vi "Main Page.vi"(8 "error in (no error)":errorcluster, 11 "Node Ptr":T1 format="%.0x") -> (0 "error out":errorcluster)   [LabVIEW 2015, in "Waveform-Processing-Custom-Device System Explorer.lvlib"]
uses:
  Waveform-Processing-Custom-Device System Explorer.lvlib
  <vilib>/NI Veristand/Custom Device API/Custom Device Item Ref.ctl
  Shared/Types/FG Action.ctl
  Types/UI Refs Ctl.ctl
  Shared/Constants.vi
  <vilib>/NI Veristand/Custom Device API/Set Item Property (Boolean).vi
  <vilib>/NI VeriStand/Custom Device API/Custom Device API.lvlib
  Shared/Waveform-Processing-Custom-Device Shared.lvlib
  Shared/Running Average/Running Average.lvlib
  Shared/Single Point/SinglePoint.lvlib
  Shared/Scaled Waveform/Scaled Waveform.lvlib
panel:
  in  "Scaled Waveform":bool
  in  "Header 2":cluster{"Section Name":string}={"Section Name"="Custom Device Item Settings"}
  out "Task Rate (Hz)":dbl
  in  "Buffer Length (s)":dbl format="%#_6f"
  out "Buffer Length (samples)":u32
  in  "Description":string
  in  "Remove Channel":bool
  in  "Add Channel":bool
  in  "Selected Waveforms":i32[](listbox)
  in  "Waveform Task":u16(ring) items=["Waveform1"=11, "Waveform2"=15]
  in  "Available Waveforms":i32[](listbox)
  in  "Single-point":bool
  in  "Running Average":bool
  in  "Header":cluster{"Section Name":string}={"Section Name"="Custom Device Item Settings"}
  in  "Name":string
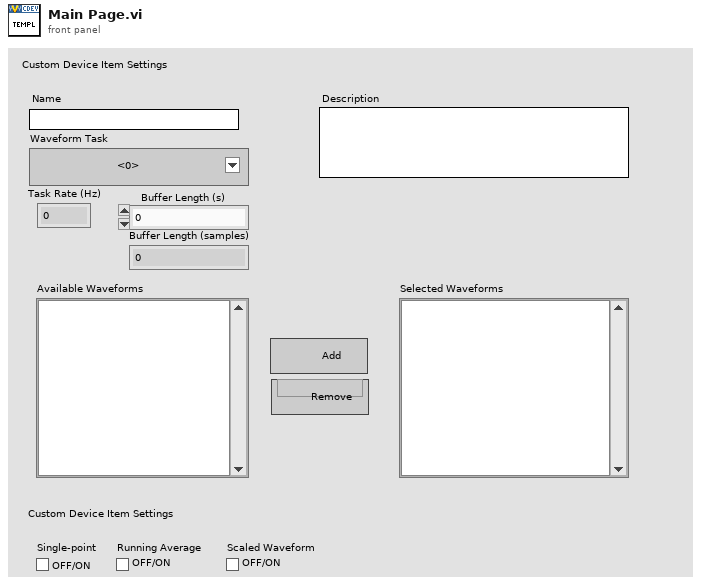
[diagram p1: front panel]
types:
  T1 = typedef "Custom Device API.lvlib/Custom Device Item Ref.ctl" = u64
  T2 = typedef "Waveform-Processing-Custom-Device Shared.lvlib/UI Refs Ctl.ctl" = cluster{"Selected Waveforms":refnum<vi>, "Available Waveforms":refnum<vi>, "Wfm Task Rate (Hz)":refnum<vi>, "Buffer Length (s)":refnum<vi>, "Buffer Length (samples)":refnum<vi>, "Add Channel":refnum<vi>, "Remove Channel":refnum<vi>, "Running Average":refnum<vi>, "Single-point":refnum<vi>, "Waveform Task":refnum<vi>, "Scaled Waveform":refnum<vi>}
  T3 = typedef "Waveform-Processing-Custom-Device Shared.lvlib/FG Action.ctl" = enum8{"GET", "SET"}
  T4 = typedef "Custom Device API.lvlib/Custom Device Item Info.ctl" = cluster{"Name":string, "Is Channel":bool, "GUID":string, "Is Waveform":bool}
  T5 = typedef "Waveform-Processing-Custom-Device Shared.lvlib/Custom Device Settings.ctl" = cluster{"CD Task Dependency":T1, "CD Task Dependency Ref":T1, "CD Task Available Wfms":string[], "CD Task Selected Wfms":string[], "Buffer Length (s)":dbl, "Buffer Length (samples)":u32, "Task Rate":dbl, "Single-point Enabled":bool, "Running Average Enabled":bool, "Scaled Waveform Enabled":bool}
  T6 = typedef "Custom Device API.lvlib/Custom Device Commands.ctl" = enum16{"Default", "Item renamed", "Shutdown", "Dynamic button pressed"}
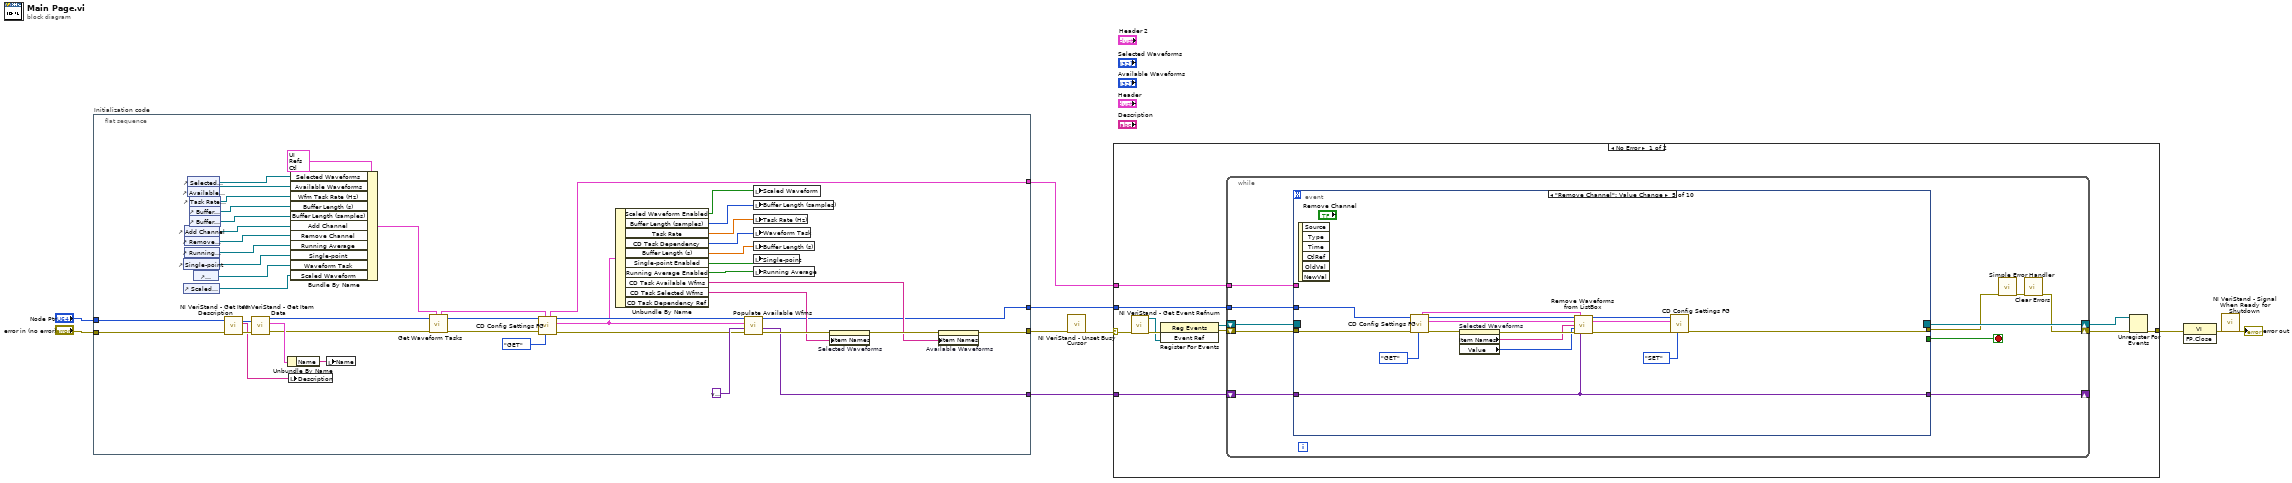
[diagram p0: block diagram]
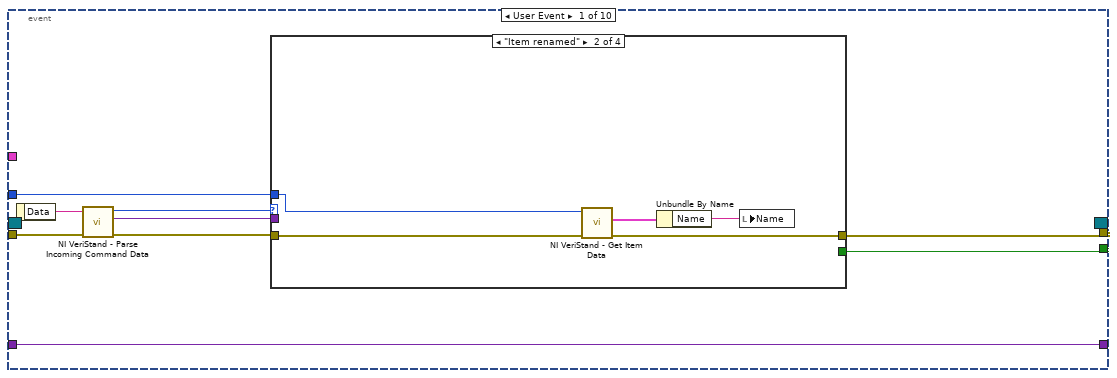
[diagram p2: hidden frame]
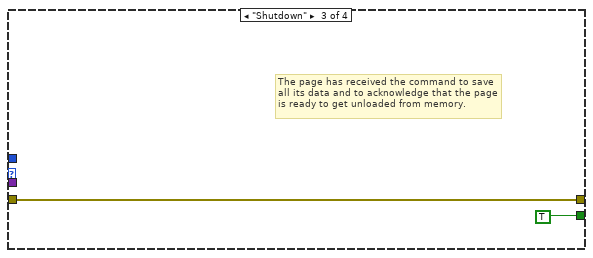
[diagram p4: hidden frame]
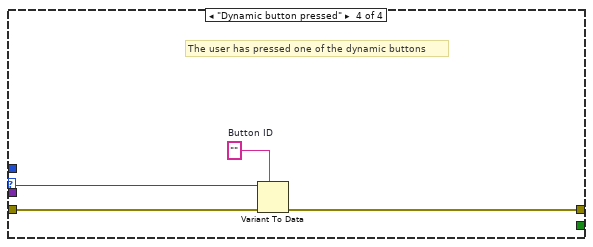
[diagram p5: hidden frame]
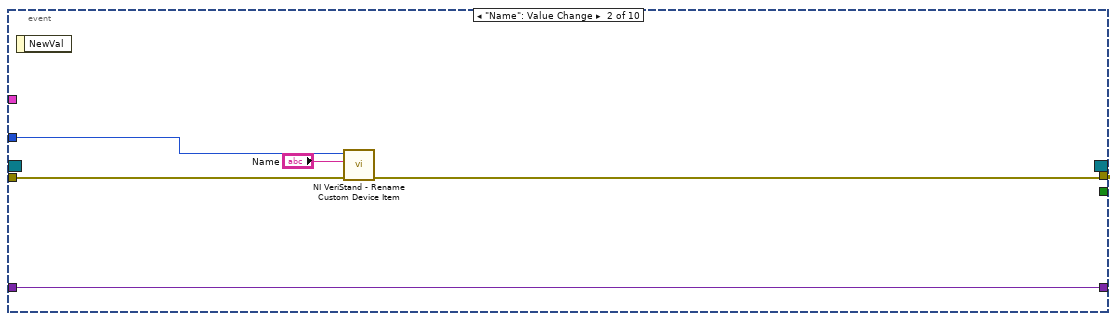
[diagram p6: hidden frame]
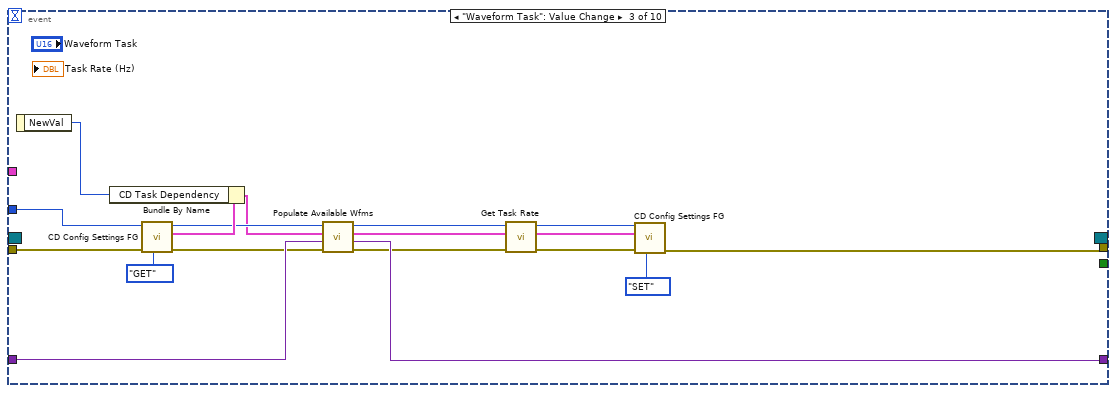
[diagram p7: hidden frame]
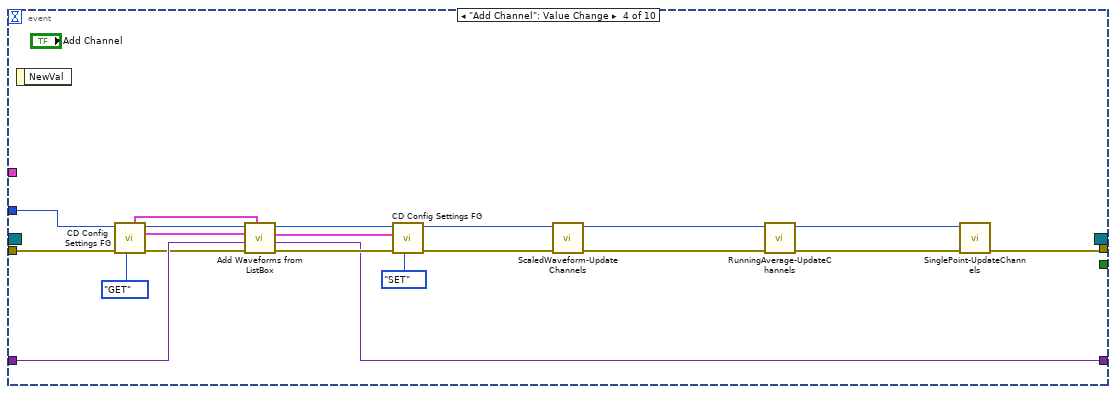
[diagram p8: hidden frame]
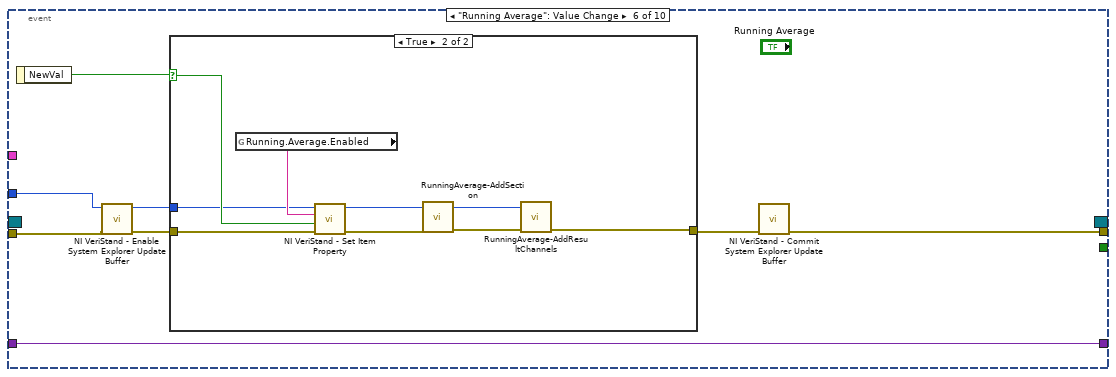
[diagram p9: hidden frame]
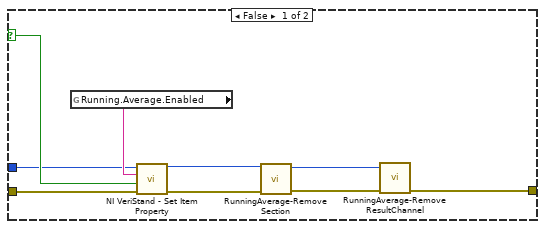
[diagram p10: hidden frame]
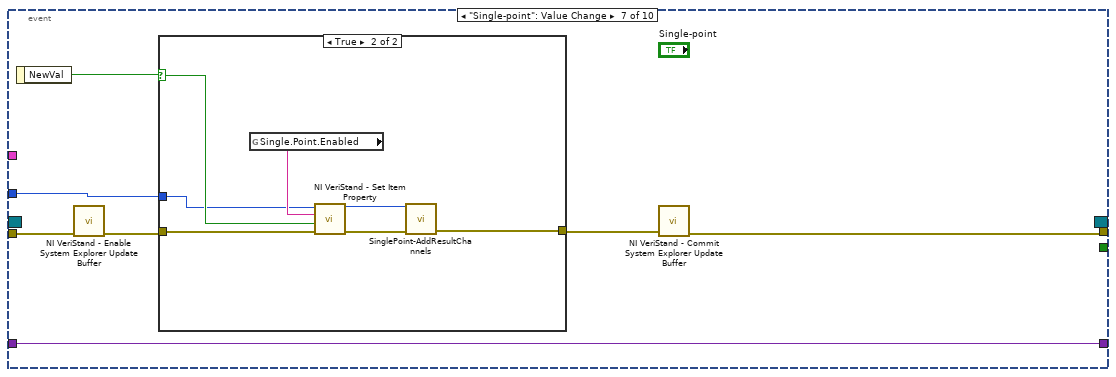
[diagram p11: hidden frame]
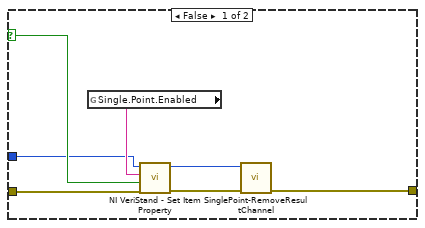
[diagram p12: hidden frame]
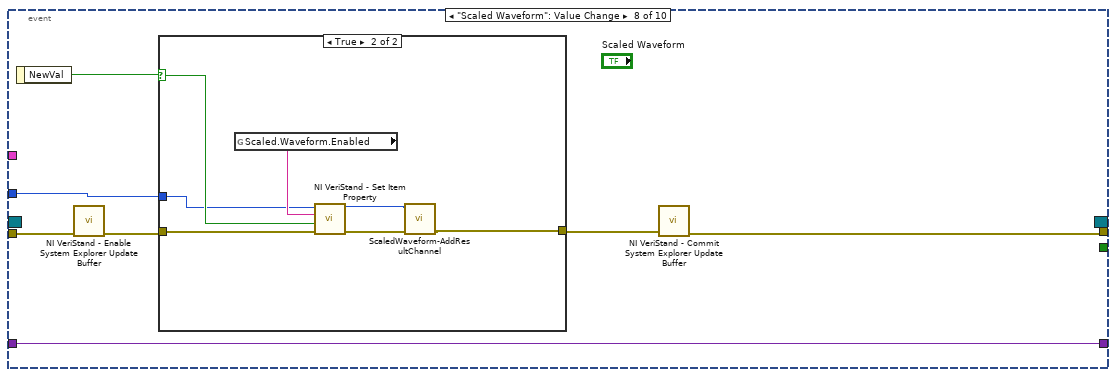
[diagram p13: hidden frame]
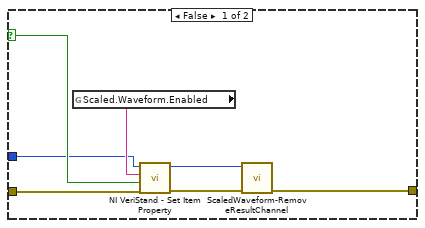
[diagram p14: hidden frame]
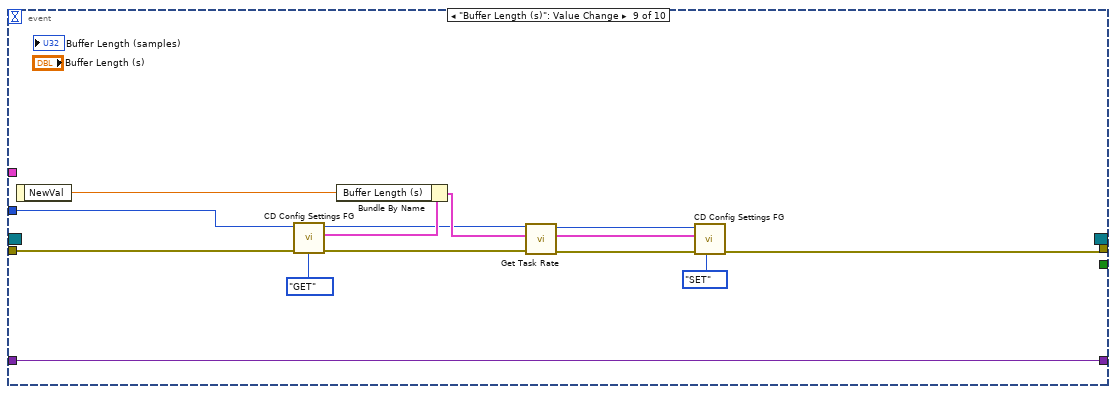
[diagram p15: hidden frame]
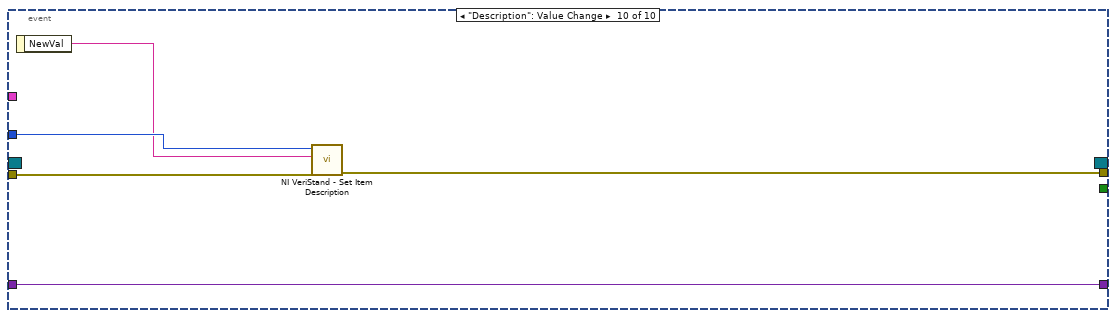
[diagram p16: hidden frame]
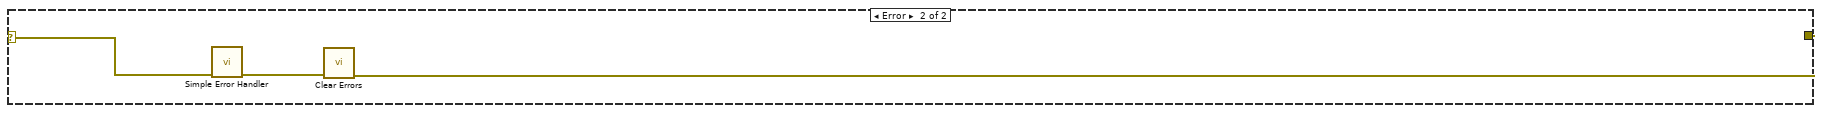
[diagram p17: hidden frame]
diagram:
  n1 = flat-sequence "Initialization code" {
    tunnel: "error in (no error)" -> [w54]
    tunnel: "Node Ptr" -> [w53]
    tunnel: [w40] -> w1
    tunnel: [w17] -> w4
    tunnel: [w15] -> w3
    tunnel: [w18] -> w2
    frame #0 {
      n2 = control-ref of="Single-point"() -> (w37:refnum<vi>)
      n3 = control-ref of="Scaled Waveform"() -> (w12:refnum<vi>)
      n4 = control-ref of="Add Channel"() -> (w34:refnum<vi>)
      n5 = control-ref of="Remove Channel"() -> (w35:refnum<vi>)
      n6 = control-ref of="Running Average"() -> (w36:refnum<vi>)
      n7 = control-ref of="Selected Waveforms"() -> (w29:refnum<vi>)
      n8 = control-ref of="Available Waveforms"() -> (w30:refnum<vi>)
      n9 = control-ref of="Task Rate (Hz)"() -> (w31:refnum<vi>)
      n10 = control-ref of="Buffer Length (s)"() -> (w32:refnum<vi>)
      n11 = control-ref of="Buffer Length (samples)"() -> (w33:refnum<vi>)
      n12 = control-ref of="Waveform Task"() -> (w19:refnum<vi>)
      n13 = call <vilib>:"NI VeriStand - Get Item Description.vi"("error in (no error)"=w54, "Item Ref in"=w53) -> ("error out"=w52:errorcluster, "Description"=w49:string, "Item Ref out"=w55:T1)  [unwired: 7 out]
      n14 = call <vilib>:"NI VeriStand - Get Item Data.vi"("error in (no error)"=w52, "Item Ref in"=w55) -> ("error out"=w26:errorcluster, "Item Info"=w51:T4, "Item Ref out"=w20:T1)  [unwired: 7 out]
      n15 = Unbundle By Name(w51) -> ("Name"=w50:string)
      n16 = local write "Description"(w49) -> ()
      n17 = Bundle By Name(cluster=T2 {"Selected Waveforms"=refnum, "Available Waveforms"=refnum, "Wfm Task Rate (Hz)"=refnum, "Buffer Length (s)"=refnum, "Buffer Length (samples)"=refnum, "Add Channel"=refnum, "Remove Channel"=refnum, "Running Average"=refnum, "Single-point"=refnum, "Waveform Task"=refnum, "Scaled Waveform"=refnum} ("UI Refs"), "Selected Waveforms"=w29, "Available Waveforms"=w30, "Wfm Task Rate (Hz)"=w31, "Buffer Length (s)"=w32, "Buffer Length (samples)"=w33, "Add Channel"=w34, "Remove Channel"=w35, "Running Average"=w36, "Single-point"=w37, "Waveform Task"=w19, "Scaled Waveform"=w12) -> (w25:T2)
      n18 = local write "Name"(w50) -> ()
      n19 = call "Get Waveform Tasks.vi"("Custom Device ref in"=w20, "error in"=w26, "UI Refs in"=w25) -> ("UI Refs out"=w24:T2, "Custom Device ref out"=w23:T1, "error out"=w27:errorcluster)  [unwired: 5 in]
      n20 = call "CD Config Settings FG.vi"("Action"=FG_Action."GET", "UI Refs"=w24, "error in (no error)"=w27, "Item Ref"=w23) -> ("error out"=w22:errorcluster, "CD Settings out"=w13:T5, "Item Ref out"=w21:T1, "UI Refs out"=w18:T2)  [unwired: 4 in]
      n21 = Unbundle By Name(w13) -> ("Scaled Waveform Enabled"=w11:bool, "Buffer Length (samples)"=w14:u32, "Task Rate"=w16:dbl, "CD Task Dependency"=w28:T1, "Buffer Length (s)"=w46:dbl, "Single-point Enabled"=w48:bool, "Running Average Enabled"=w47:bool, "CD Task Available Wfms"=w41:string[], "CD Task Selected Wfms"=w42:string[])  [unwired: 1 out]
      n22 = call "Populate Available Wfms.vi"("error in"=w22, "ListBox Variant"=variant, "CD Settings"=w13, "CustomDevice Ref"=w21) -> ("error out"=w44:errorcluster, "ListBox Variant"=w40:variant, "CustomDevice Ref"=w15:T1)  [unwired: 4 in, 1 out]
      n23 = local write "Scaled Waveform"(w11) -> ()
      n24 = local write "Buffer Length (samples)"(w14) -> ()
      n25 = local write "Task Rate (Hz)"(w16) -> ()
      n26 = local write "Waveform Task"(w28) -> ()
      n27 = local write "Buffer Length (s)"(w46) -> ()
      n28 = local write "Single-point"(w48) -> ()
      n29 = local write "Running Average"(w47) -> ()
      n30 = property on="Selected Waveforms" class="LstBox (strict)"(error in=w44, "Item Names"=w42) -> (error out=w43:errorcluster)  [unwired: 1 in, 1 out]
      n31 = property on="Available Waveforms" class="LstBox (strict)"(error in=w43, "Item Names"=w41) -> (error out=w17:errorcluster)  [unwired: 1 in, 1 out]
    }
  }
  n32 = call <vilib>:"NI VeriStand - Unset Busy Cursor.vi"("error in (no error)"=w4) -> ("error out"=w6:errorcluster)  [unwired: 10 out]
  n33 = case shown="No Error" w6 {
    selector: w6 -> [w59 w246]
    tunnel: [w63 w244] -> w10
    tunnel: w3 -> [w58 _]
    tunnel: w1 -> [w57 _]
    tunnel: w2 -> [w56 _]
    frame No Error {
      n34 = call <vilib>:"NI VeriStand - Get Event Refnum.vi"("error in (no error)"=w59) -> ("error out"=w66:errorcluster, "Event Ref"=w62:refnum<user-event>)  [unwired: 9 out]
      n35 = register-events(error in=w66, w62) -> (reference out=w60:refnum<event-registration>, error out=w61:errorcluster)  [unwired: 1 in]
      n36 = while {
        shift-right: [w73] -> w64
        shift-left: w61 -> [w69]
        shift-right: [w77] -> w65
        shift-left: w60 -> [w76]
        tunnel: w58 -> [w72]
        shift-right: [w71] -> _
        shift-left: w57 -> [w70]
        tunnel: w56 -> [w67]
        stop <- w75 stop-if-true
        n37 = event shown="[4] \"Remove Channel\": Value Change" {
          selector: w76 -> [_ _ _ _ _ _ _ _ _ _]
          dyn-events: [_ _ _ _ _ _ _ _ _ _] -> w77
          timeout: _ -> [_ _ _ _ _ _ _ _ _ _]
          tunnel: w69 -> [w86 w103 w118 w135 w154 w161 w186 w207 w237 w243]
          tunnel: [w82 _ _ _ _ _ _ _ _ _] -> w75
          tunnel: [w81 w102 w104 w131 w143 w158 w183 w204 w225 w242] -> w68
          tunnel: w72 -> [w79 w100 w117 w141 w157 w163 w188 w209 w235 w241]
          tunnel: [w78 w99 w121 w127 w142 w162 w187 w208 w238 w239] -> w71
          tunnel: w70 -> [w78 w99 w120 w129 w142 w162 w187 w208 w238 w239]
          tunnel: w67 -> [_ _ _ _ _ _ _ _ _ _]
          event User Event {
            n38 = event-data() -> ("Data"=w85:string)  [unwired: 1 out]
            n39 = call <vilib>:"NI VeriStand - Parse Incoming Command Data.vi"("error in (no error)"=w86, "Incoming data"=w85) -> ("error out"=w84:errorcluster, "Outgoing data"=w80:variant, "Action"=w83:T6)  [unwired: 7 out]
            n40 = case shown="\"Item renamed\"" w83 {
              tunnel: w84 -> [w87 w92 w93 w98]
              tunnel: [_ _ TRUE _] -> w82
              tunnel: [w87 w90 w93 w95] -> w81
              tunnel: w80 -> [_ _ _ w97]
              tunnel: w79 -> [_ w88 _ _]
              frame "Default", Default {
              }
              frame "Item renamed" {
                n41 = call <vilib>:"NI VeriStand - Get Item Data.vi"("error in (no error)"=w92, "Item Ref in"=w88) -> ("error out"=w90:errorcluster, "Item Info"=w91:T4)  [unwired: 8 out]
                n42 = Unbundle By Name(w91) -> ("Name"=w89:string)
                n43 = local write "Name"(w89) -> ()
              }
              frame "Shutdown" {
                # "The page has received the command to save all its data and to acknowledge that the page is ready to get unloaded from memory."
              }
              frame "Dynamic button pressed" {
                w96 = ""  # Button ID
                # "The user has pressed one of the dynamic buttons"
                n44 = Variant To Data(error in=w98, type=w96, Variant=w97) -> (error out=w95:errorcluster)  [unwired: 1 out]
              }
            }
          }
          event "Name": Value Change {
            n45 = event-data() -> ()  [unwired: 2 out]
            n46 = call <vilib>:"NI VeriStand - Rename Custom Device Item.vi"("error in (no error)"=w103, "New Name"="Name", "Item Ref in"=w100) -> ("error out"=w102:errorcluster)  [unwired: 1 in, 7 out]
          }
          event "Waveform Task": Value Change {
            n47 = event-data() -> ("NewVal"=w119:u16)  [unwired: 1 out]
            n48 = call "CD Config Settings FG.vi"("Action"=FG_Action."GET", "error in (no error)"=w118, "Item Ref"=w117) -> ("error out"=w113:errorcluster, "CD Settings out"=w116:T5, "Item Ref out"=w112:T1)  [unwired: 5 in, 1 out]
            n49 = Bundle By Name(cluster=w116, "CD Task Dependency"=w119) -> (w111:T5)
            n50 = call "Populate Available Wfms.vi"("error in"=w113, "ListBox Variant"=w120, "CD Settings"=w111, "CustomDevice Ref"=w112) -> ("error out"=w110:errorcluster, "ListBox Variant"=w121:variant, "CD Settings out"=w109:T5, "CustomDevice Ref"=w108:T1)  [unwired: 4 in]
            n51 = call "Get Task Rate.vi"("error in"=w110, "CD Settings"=w109, "CustomDevice Ref"=w108) -> ("error out"=w106:errorcluster, "CD Settings out"=w105:T5, "CustomDevice Ref out"=w107:T1)  [unwired: 6 in]
            n52 = call "CD Config Settings FG.vi"("Action"=FG_Action."SET", "error in (no error)"=w106, "CD Settings in"=w105, "Item Ref"=w107) -> ("error out"=w104:errorcluster)  [unwired: 4 in, 3 out]
          }
          event "Add Channel": Value Change {
            n53 = event-data() -> ()  [unwired: 2 out]
            n54 = call "CD Config Settings FG.vi"("Action"=FG_Action."GET", "error in (no error)"=w135, "Item Ref"=w141) -> ("error out"=w128:errorcluster, "CD Settings out"=w137:T5, "Item Ref out"=w134:T1, "UI Refs out"=w126:T2)  [unwired: 5 in]
            n55 = call "Add Waveforms from ListBox.vi"("UI Refs"=w126, "error in (no error)"=w128, "Wfm Ref LUT"=w129, "CD Settings in"=w137, "Custom Device Ref in"=w134) -> ("error out"=w140:errorcluster, "Wfm Ref LUT out"=w127:variant, "CD Settings out"=w136:T5, "Custom Device Ref out"=w133:T1)  [unwired: 1 in]
            n56 = call "CD Config Settings FG.vi"("Action"=FG_Action."SET", "error in (no error)"=w140, "CD Settings in"=w136, "Item Ref"=w133) -> ("error out"=w123:errorcluster, "Item Ref out"=w125:T1)  [unwired: 4 in, 2 out]
            n57 = call "ScaledWaveform-UpdateChannels.vi"("Error in"=w123, "Custom Device ref in"=w125) -> ("Error out"=w122:errorcluster, "Custom Device ref out"=w124:T1)  [unwired: 8 in]
            n58 = call "RunningAverage-UpdateChannels.vi"("Error in"=w122, "Custom Device ref in"=w124) -> ("Error out"=w132:errorcluster, "Custom Device ref out"=w130:T1)  [unwired: 8 in]
            n59 = call "SinglePoint-UpdateChannels.vi"("Error in"=w132, "Custom Device ref in"=w130) -> ("Error out"=w131:errorcluster)  [unwired: 8 in, 1 out]
          }
          event "Remove Channel": Value Change {
            n60 = event-data() -> ()  [unwired: 7 out]
            n61 = call "CD Config Settings FG.vi"("Action"=FG_Action."GET", "error in (no error)"=w154, "Item Ref"=w157) -> ("error out"=w153:errorcluster, "CD Settings out"=w148:T5, "Item Ref out"=w147:T1, "UI Refs out"=w146:T2)  [unwired: 5 in]
            n62 = property on="Selected Waveforms" class="LstBox (strict)"(error in=w153) -> (error out=w152:errorcluster, "Item Names"=w149:string[], "Value"=w150:i32[])  [unwired: 1 in, 1 out]
            n63 = call "Remove Waveforms from ListBox.vi"("Custom Device Ref in"=w147, "UI Refs"=w146, "CD Settings in"=w148, "Item Names"=w149, "Value"=w150, "error in (no error)"=w152, "Waveform Ref LUT"=w142) -> ("Custom Device Ref out"=w145:T1, "CD Settings out"=w144:T5, "error out"=w151:errorcluster)  [unwired: 6 in]
            n64 = call "CD Config Settings FG.vi"("Action"=FG_Action."SET", "error in (no error)"=w151, "CD Settings in"=w144, "Item Ref"=w145) -> ("error out"=w143:errorcluster)  [unwired: 4 in, 3 out]
          }
          event "Running Average": Value Change {
            n65 = event-data() -> ("NewVal"=w164:bool)  [unwired: 1 out]
            n66 = call <vilib>:"NI VeriStand - Enable System Explorer Update Buffer.vi"("error in (no error)"=w161) -> ("error out"=w160:errorcluster)  [unwired: 10 in]
            n67 = case shown="True" w164 {
              selector: w164 -> [w171 w181]
              tunnel: w160 -> [w173 w174]
              tunnel: [w166 w175] -> w159
              tunnel: w163 -> [w170 w178]
              frame False {
                n68 = global read "Constants.vi" "Running.Average.Enabled"() -> (w172:string)
                n69 = call-poly <vilib>:"NI VeriStand - Set Item Property.vi"("error in (no error)"=w173, "Value"=w171, "Property Name"=w172, "Item Ref in"=w170) -> ("error out"=w168:errorcluster, "Item Ref out"=w169:T1)  [unwired: 5 in, 1 out]
                n70 = call "RunningAverage-RemoveSection.vi"("Error in"=w168, "Custom Device ref"=w169) -> ("Error out"=w167:errorcluster, "Custom Device ref out"=w165:T1)  [unwired: 8 in]
                n71 = call "RunningAverage-RemoveResultChannel.vi"("Error in"=w167, "Custom Device ref"=w165) -> ("Error out"=w166:errorcluster)  [unwired: 8 in, 1 out]
              }
              frame True {
                n72 = global read "Constants.vi" "Running.Average.Enabled"() -> (w182:string)
                n73 = call-poly <vilib>:"NI VeriStand - Set Item Property.vi"("error in (no error)"=w174, "Value"=w181, "Property Name"=w182, "Item Ref in"=w178) -> ("error out"=w180:errorcluster, "Item Ref out"=w179:T1)  [unwired: 5 in, 1 out]
                n74 = call "RunningAverage-AddSection.vi"("Error in"=w180, "Custom Device ref"=w179) -> ("Error out"=w177:errorcluster, "Custom Device ref out"=w176:T1)  [unwired: 8 in]
                n75 = call "RunningAverage-AddResultChannels.vi"("Error in"=w177, "Custom Device ref"=w176) -> ("Error out"=w175:errorcluster)  [unwired: 8 in, 1 out]
              }
            }
            n76 = call <vilib>:"NI VeriStand - Commit System Explorer Update Buffer.vi"("error in (no error)"=w159) -> ("error out"=w158:errorcluster)  [unwired: 10 in]
          }
          event "Single-point": Value Change {
            n77 = event-data() -> ("NewVal"=w189:bool)  [unwired: 1 out]
            n78 = call <vilib>:"NI VeriStand - Enable System Explorer Update Buffer.vi"("error in (no error)"=w186) -> ("error out"=w185:errorcluster)  [unwired: 10 in]
            n79 = case shown="True" w189 {
              selector: w189 -> [w195 w201]
              tunnel: w185 -> [w191 w202]
              tunnel: [w190 w198] -> w184
              tunnel: w188 -> [w192 w197]
              frame False {
                n80 = global read "Constants.vi" "Single.Point.Enabled"() -> (w196:string)
                n81 = call-poly <vilib>:"NI VeriStand - Set Item Property.vi"("error in (no error)"=w191, "Value"=w195, "Property Name"=w196, "Item Ref in"=w192) -> ("error out"=w194:errorcluster, "Item Ref out"=w193:T1)  [unwired: 5 in, 1 out]
                n82 = call "SinglePoint-RemoveResultChannel.vi"("Error in"=w194, "Custom Device ref"=w193) -> ("Error out"=w190:errorcluster)  [unwired: 8 in, 1 out]
              }
              frame True {
                n83 = global read "Constants.vi" "Single.Point.Enabled"() -> (w203:string)
                n84 = call-poly <vilib>:"NI VeriStand - Set Item Property.vi"("error in (no error)"=w202, "Value"=w201, "Property Name"=w203, "Item Ref in"=w197) -> ("error out"=w200:errorcluster, "Item Ref out"=w199:T1)  [unwired: 5 in, 1 out]
                n85 = call "SinglePoint-AddResultChannels.vi"("Error in"=w200, "Custom Device ref"=w199) -> ("Error out"=w198:errorcluster)  [unwired: 8 in, 1 out]
              }
            }
            n86 = call <vilib>:"NI VeriStand - Commit System Explorer Update Buffer.vi"("error in (no error)"=w184) -> ("error out"=w183:errorcluster)  [unwired: 10 in]
          }
          event "Scaled Waveform": Value Change {
            n87 = event-data() -> ("NewVal"=w210:bool)  [unwired: 1 out]
            n88 = call <vilib>:"NI VeriStand - Enable System Explorer Update Buffer.vi"("error in (no error)"=w207) -> ("error out"=w206:errorcluster)  [unwired: 10 in]
            n89 = case shown="True" w210 {
              selector: w210 -> [w216 w222]
              tunnel: w206 -> [w214 w223]
              tunnel: [w211 w218] -> w205
              tunnel: w209 -> [w215 w221]
              frame False {
                n90 = global read "Constants.vi" "Scaled.Waveform.Enabled"() -> (w217:string)
                n91 = call-poly <vilib>:"NI VeriStand - Set Item Property.vi"("error in (no error)"=w214, "Value"=w216, "Property Name"=w217, "Item Ref in"=w215) -> ("error out"=w213:errorcluster, "Item Ref out"=w212:T1)  [unwired: 5 in, 1 out]
                n92 = call "ScaledWaveform-RemoveResultChannel.vi"("Error in"=w213, "Custom Device ref"=w212) -> ("Error out"=w211:errorcluster)  [unwired: 8 in, 1 out]
              }
              frame True {
                n93 = global read "Constants.vi" "Scaled.Waveform.Enabled"() -> (w224:string)
                n94 = call-poly <vilib>:"NI VeriStand - Set Item Property.vi"("error in (no error)"=w223, "Value"=w222, "Property Name"=w224, "Item Ref in"=w221) -> ("error out"=w220:errorcluster, "Item Ref out"=w219:T1)  [unwired: 5 in, 1 out]
                n95 = call "ScaledWaveform-AddResultChannel.vi"("Error in"=w220, "Custom Device ref"=w219) -> ("Error out"=w218:errorcluster)  [unwired: 8 in, 1 out]
              }
            }
            n96 = call <vilib>:"NI VeriStand - Commit System Explorer Update Buffer.vi"("error in (no error)"=w205) -> ("error out"=w204:errorcluster)  [unwired: 10 in]
          }
          event "Buffer Length (s)": Value Change {
            n97 = event-data() -> ("NewVal"=w233:dbl)  [unwired: 1 out]
            n98 = call "CD Config Settings FG.vi"("Action"=FG_Action."GET", "error in (no error)"=w237, "Item Ref"=w235) -> ("error out"=w231:errorcluster, "CD Settings out"=w234:T5, "Item Ref out"=w230:T1)  [unwired: 5 in, 1 out]
            n99 = Bundle By Name(cluster=w234, "Buffer Length (s)"=w233) -> (w232:T5)
            n100 = call "Get Task Rate.vi"("error in"=w231, "CD Settings"=w232, "CustomDevice Ref"=w230) -> ("error out"=w229:errorcluster, "CD Settings out"=w227:T5, "CustomDevice Ref out"=w228:T1)  [unwired: 6 in]
            n101 = call "CD Config Settings FG.vi"("Action"=FG_Action."SET", "error in (no error)"=w229, "CD Settings in"=w227, "Item Ref"=w228) -> ("error out"=w225:errorcluster)  [unwired: 4 in, 3 out]
          }
          event "Description": Value Change {
            n102 = event-data() -> ("NewVal"=w240:string)  [unwired: 1 out]
            n103 = call <vilib>:"NI VeriStand - Set Item Description.vi"("error in (no error)"=w243, "Description"=w240, "Item Ref in"=w241) -> ("error out"=w242:errorcluster)  [unwired: 8 out]
          }
        }
        n104 = call <vilib>:"Simple Error Handler.vi"("error in (no error)"=w68) -> ("error out"=w74:errorcluster)  [unwired: 1 in, 7 out]
        n105 = call <vilib>:"Clear Errors.vi"("error in (no error)"=w74) -> ("error out"=w73:errorcluster)  [unwired: 1 in, 5 out]
      }
      n106 = Unregister For Events(event registration refnum=w65, error in=w64) -> (error out=w63:errorcluster)
    }
    frame Error {
      n107 = call <vilib>:"Simple Error Handler.vi"("error in (no error)"=w246) -> ("error out"=w245:errorcluster)  [unwired: 1 in, 7 out]
      n108 = call <vilib>:"Clear Errors.vi"("error in (no error)"=w245) -> ("error out"=w244:errorcluster)  [unwired: 1 in, 5 out]
    }
  }
  n109 = invoke class="VI" method="FP.Close"(error in=w10) -> (error out=w9:errorcluster)  [unwired: 2 in, 2 out]
  n110 = call <vilib>:"NI VeriStand - Signal When Ready for Shutdown.vi"("error in (no error)"=w9) -> ("error out"=→"error out":errorcluster)  [unwired: 10 out]
